vi "logForceActuatorTest.vi"(8 "error in (no error)":errorcluster, 10 "EventForceActuatorTest":T1, 11 "M1M3SAL in":refnum<class "M1M3SAL.lvclass">) -> (0 "error out":errorcluster, 3 "M1M3SAL out":refnum<class "M1M3SAL.lvclass">)   [LabVIEW 2016, in "M1M3SupportCommunicator.lvlib" / "M1M3SAL.lvclass"]
uses:
  M1M3SAL.lvclass
  DataTypes/Topics/EventForceActuatorTest.ctl
  DataTypes/Topics/Parts/Timestamp.ctl
  DataTypes/Topics/Parts/TestStatus.ctl
  DataTypes/MessageHeader.ctl
  DataTypes/MessageTypes.ctl
  DataTypes/MessageTopics.ctl
  M1M3SAL.lvclass/M1M3SAL.ctl
  writeU8.vi
  M1M3SupportCommunicator.lvlib
  DataTypes/Topics/M1M3SupportTopics.lvlib
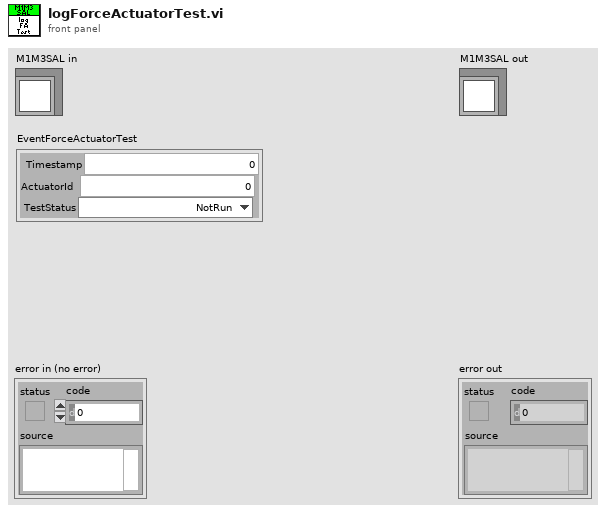
[diagram p1: front panel]
types:
  T1 = typedef "M1M3SupportTopics.lvlib/EventForceActuatorTest.ctl" = cluster{"Timestamp":T2, "ActuatorId":i32, "TestStatus":T3}
  T2 = typedef "M1M3SupportTopics.lvlib/Timestamp.ctl" = dbl
  T3 = typedef "M1M3SupportTopics.lvlib/TestStatus.ctl" = enum16{"NotRun", "Pass", "Fail"}
  T4 = typedef "M1M3SupportCommunicator.lvlib/MessageHeader.ctl" = cluster{"Type":T5, "Topic":T6, "Size":i32}
  T5 = typedef "M1M3SupportCommunicator.lvlib/MessageTypes.ctl" = enum8{"None", "PutSample", "GetNextSample", "LogEvent", "GetEvent", "IssueCommand", "CommandId", "WaitForCompletion", "AcceptCommand", "AckCommand"}
  T6 = typedef "M1M3SupportCommunicator.lvlib/MessageTopics.ctl" = enum8{"None", "ForceActuatorData", "MirrorForceData", "HardpointData", "AirData", "DynamicData", "FPGAData", "IMSData", "ForceActuatorStatus", "ElevationData", "HardpointStatus", "HardpointActuatorChase", "AirStatus", "ForceActuatorSafetyChecks", "ForceActuatorTest", "ActuatorBroadcastCounter", "StatusChecks", "CellChecks", "HardpointActuatorBreakaway", "RaiseMirrorComplete", "ILCCommunication", "ElevationAngleChecks", "DetailedState", "ServoLoops", "ForceActuatorInfo", "LowerMirrorComplete", "HardpointActuatorInfo", "SettingsApplied", "ErrorCode", "StartupChecks", "SummaryState", "SettingVersions", "ActuatorTestStatus", "AppliedSettingsMatchStart", "Enable", "EnterMaintenance", "Standby", "AbortLowerM1M3", "ApplyAberrationByForces", "ApplyAOSCorrectionByBendingModes", "ClearAOSCorrection", "Start", "RaiseM1M3", "TestForceActuator", "LowerM1M3", "ApplyAOSCorrectionByForces", "Disable", "ApplyAberationByBendingMode", "TestHardpoint", "ManipulateM1M3", "ClearAberration", "Exit", "TestAir", "AbortRaiseM1M3", "MoveHardpointActuators", "ExitMaintenance", "Shutdown"}
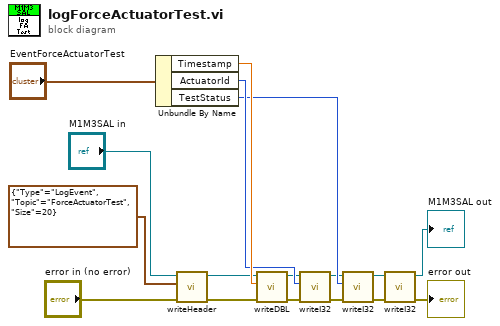
[diagram p0: block diagram]
diagram:
  n1 = Unbundle By Name("EventForceActuatorTest") -> ("Timestamp"=w14:T2, "ActuatorId"=w13:i32, "TestStatus"=w12:T3)
  n2 = call "writeHeader.vi"("error in (no error)"="error in (no error)", "MessageHeader"=T4 {"Type"=enum."LogEvent", "Topic"=enum."ForceActuatorTest", "Size"=20}, "M1M3SAL in"="M1M3SAL in") -> ("error out"=w6:errorcluster, "M1M3SAL out"=w11:refnum<class "M1M3SAL.lvclass">)  [unwired: 7 in]
  n3 = call "writeDBL.vi"("error in (no error)"=w6, "Input"=w14, "M1M3SAL in"=w11) -> ("error out"=w5:errorcluster, "M1M3SAL out"=w10:refnum<class "M1M3SAL.lvclass">)  [unwired: 7 in]
  n4 = call "writeI32.vi"("error in (no error)"=w5, "Input"=w13, "M1M3SAL in"=w10) -> ("error out"=w4:errorcluster, "M1M3SAL out"=w9:refnum<class "M1M3SAL.lvclass">)  [unwired: 7 in]
  n5 = call "writeI32.vi"("error in (no error)"=w4, "Input"=w12, "M1M3SAL in"=w9) -> ("error out"=w3:errorcluster, "M1M3SAL out"=w8:refnum<class "M1M3SAL.lvclass">)  [unwired: 7 in]
  n6 = call "writeI32.vi"("error in (no error)"=w3, "M1M3SAL in"=w8) -> ("error out"=→"error out":errorcluster, "M1M3SAL out"=→"M1M3SAL out":refnum<class "M1M3SAL.lvclass">)  [unwired: 8 in]
